vi "Insert Item.vi"(0 "State In":T1={"Prompt"="Click to add", "Listbox"=refnum, "Required"={"Strings"=[], "Bottom"=FALSE, "Italic"=FALSE, "FG"=0, "BG"=16777215, "Bold"=FALSE}, "Items"=[], "Req'd"=[], "Events"={"Items Changed"=refnum, "List Changed"=refnum}, "Max Rows"=-1, "Default name"=""}, 7 "Insert at":i32) -> (4 "State Out":T1={"Prompt"="Click to add", "Listbox"=refnum, "Required"={"Strings"=[], "Bottom"=FALSE, "Italic"=FALSE, "FG"=0, "BG"=16777215, "Bold"=FALSE}, "Items"=[], "Req'd"=[], "Events"={"Items Changed"=refnum, "List Changed"=refnum}, "Max Rows"=-1, "Default name"=""})   [LabVIEW 2015, in "KListboxEx.xctl"]
uses:
  KListboxEx.xctl
  State.ctl
  Required.ctl
  Events.ctl
  Event Action.ctl
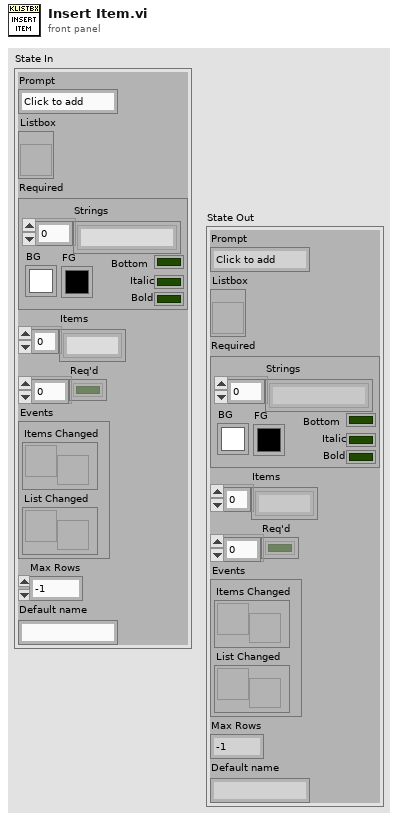
[diagram p1: front panel]
types:
  T1 = typedef "KListboxEx.xctl/State.ctl" = cluster{"Prompt":string, "Listbox":refnum<vi>, "Required":T2, "Items":string[], "Req'd":bool[], "Events":T3, "Max Rows":i32, "Default name":string}
  T2 = typedef "KListboxEx.xctl/Required.ctl" = cluster{"Strings":string[], "Bottom":bool, "Italic":bool, "FG":u32, "BG":u32, "Bold":bool}
  T3 = typedef "KListboxEx.xctl/Events.ctl" = cluster{"Items Changed":refnum<user-event>, "List Changed":refnum<user-event>}
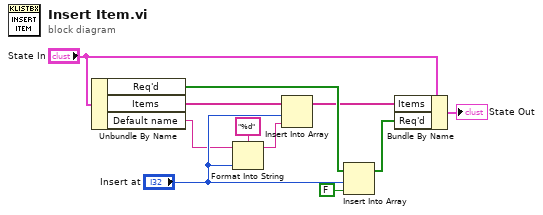
[diagram p0: block diagram]
diagram:
  n1 = Unbundle By Name("State In") -> ("Req'd"=w7:bool[], "Items"=w9:string[], "Default name"=w1:string)
  n2 = Format Into String(format string="%d", initial string=w1, "Insert at") -> (resulting string=w10:string)  [unwired: 1 in, 1 out]
  n3 = Insert Into Array(array=w9, index="Insert at", new element=w10) -> (w3:string[])
  n4 = Insert Into Array(array=w7, index="Insert at", new element=FALSE ("new element/subarray")) -> (w4:bool[])
  n5 = Bundle By Name(cluster="State In", "Items"=w3, "Req'd"=w4) -> (→"State Out":T1)
